vi "ssss.vi"() -> ()   [LabVIEW 2016]
panel:
  in  "String":string
  in  "Stop Button":bool
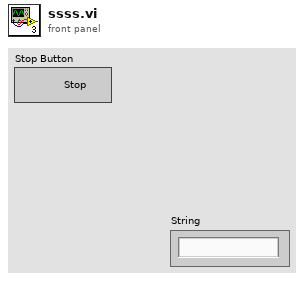
[diagram p1: front panel]
types:
  T1 = enum16{"Read", "Write", "ReadWrite", "BufferedRead", "BufferedReadWrite"}
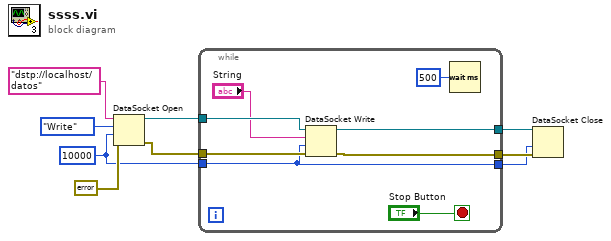
[diagram p0: block diagram]
diagram:
  w6 = 10000 ("ms timeout (10000)")
  n1 = DataSocket Open(8:errorcluster {"status"=FALSE, "code"=0, "source"=""} ("error in (no error)"), 9:w6, 10:T1."Write" ("mode"), 11:"dstp://localhost/datos" ("connection in")) -> (0:w4:errorcluster, 3:w5:refnum<k13>)
  n2 = while {
    tunnel: w6 -> [w11]
    tunnel: w5 -> [w15]
    tunnel: w4 -> [w14]
    tunnel: [w13] -> w3
    tunnel: [w12] -> w2
    tunnel: [w11] -> w1
    stop <- "Stop Button" stop-if-true
    n3 = DataSocket Write(8:w14, 9:w11, 10:"String", 11:w15) -> (0:w13:errorcluster, 3:w12:refnum<k13>)  [unwired: 1 out]
    n4 = Wait (ms)(milliseconds to wait=u32 500) -> ()  [unwired: 1 out]
  }
  n5 = DataSocket Close(8:w3, 9:w1, 11:w2) -> ()  [unwired: 2 out]
